vi "Create String3.vi"(0 "Torque FB":dbl, 1 "Torque FF":dbl, 2 "HRref":dbl, 4 "Heart Rate":u32, 5 "Tdes":dbl, 6 "Cadence":dbl, 7 "String in":string, 8 "Torque Motor":dbl, 9 "Power":dbl, 10 "Torque Rider":dbl, 11 "t0":timestamp) -> (3 "String out":string)   [LabVIEW 2013]
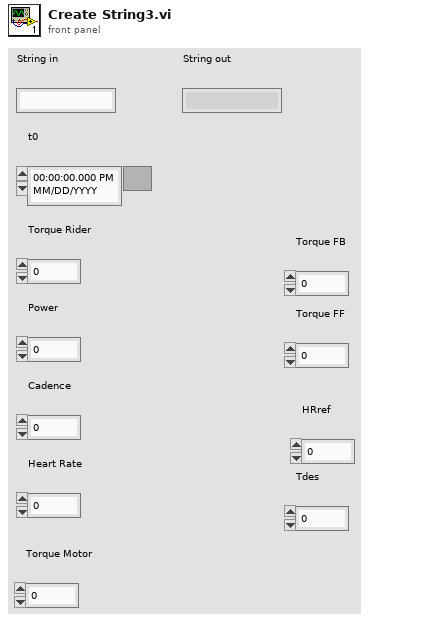
[diagram p1: front panel]
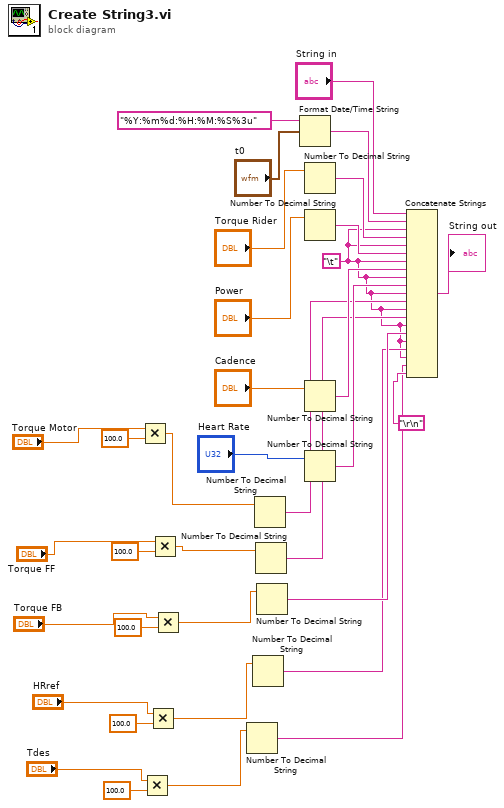
[diagram p0: block diagram]
diagram:
  w5 = "\t"
  n1 = Multiply(x="Torque Motor", y=100.0) -> (x*y=w17:dbl)
  n2 = Multiply(x="Tdes", y=100.0) -> (x*y=w3:dbl)
  n3 = Multiply(x="HRref", y=100.0) -> (x*y=w9:dbl)
  n4 = Multiply(x="Torque FF", y=100.0) -> (x*y=w14:dbl)
  n5 = Multiply(x="Torque FB", y=100.0) -> (x*y=w10:dbl)
  n6 = Number To Decimal String(number=w3) -> (decimal integer string=w1:string)  [unwired: 1 in]
  n7 = Number To Decimal String(number=w9) -> (decimal integer string=w7:string)  [unwired: 1 in]
  n8 = Number To Decimal String(number=w17) -> (decimal integer string=w22:string)  [unwired: 1 in]
  n9 = Number To Decimal String(number=w14) -> (decimal integer string=w21:string)  [unwired: 1 in]
  n10 = Number To Decimal String(number=w10) -> (decimal integer string=w20:string)  [unwired: 1 in]
  n11 = Format Date/Time String(time format string (%c)="%Y:%m%d:%H:%M:%S%3u", seconds (now)="t0") -> (date/time string=w26:string)  [unwired: 1 in]
  n12 = Number To Decimal String(number="Torque Rider") -> (decimal integer string=w29:string)  [unwired: 1 in]
  n13 = Number To Decimal String(number="Power") -> (decimal integer string=w30:string)  [unwired: 1 in]
  n14 = Number To Decimal String(number="Cadence") -> (decimal integer string=w31:string)  [unwired: 1 in]
  n15 = Number To Decimal String(number="Heart Rate") -> (decimal integer string=w35:string)  [unwired: 1 in]
  n16 = Concatenate Strings("String in", w26, w5, w29, w5, w30, w5, w31, w5, w35, w5, w22, w5, w21, w5, w20, w5, w7, w5, w1, "\r\n") -> (→"String out":string)
